vi "Read SubComponent Parameter - Raw.vi"(8 "error in (no error)":errorcluster, 10 "Parameter":string, 11 "1553 SubComponent in":refnum<class "1553 SubComponent.lvclass">) -> (0 "error out":errorcluster, 2 "Raw Data":u64 format="%016x")   [LabVIEW 2020, in "BCI-1553 API.lvlib" / "1553 SubComponent.lvclass"]
doc: "Reads a raw U64 value for a single parameter, as opposed to all the parameters at once."
uses:
  1553 SubComponent.lvclass
  Frames & Messages/TypeDefs/Parameter Table Data.ctl
  Frames & Messages/TypeDefs/Scaling Information.ctl
  1553 SubComponent.lvclass/1553 SubComponent.ctl
  Dependencies/Registry/Registry.lvclass/Registry.ctl
  Dependencies/Registry/Registry.lvclass
  BCI-1553 API.lvlib
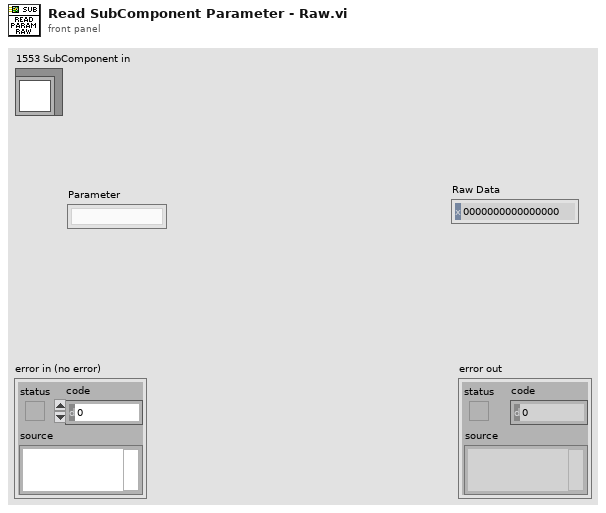
[diagram p1: front panel]
types:
  T1 = typedef "BCI-1553 API.lvlib/Parameter Table Data.ctl" = cluster{"Parameter Name":string, "Base Word":u16, "Address":u16, "Value":u64, "Mask":u16[], "Scaling Info":T2}
  T2 = typedef "BCI-1553 API.lvlib/Scaling Information.ctl" = cluster{"Bit Offset":i32, "Bit Count":i32, "LSB Resolution":dbl, "2's Complement":bool, "Big Endian":bool, "Sign Bit":bool}
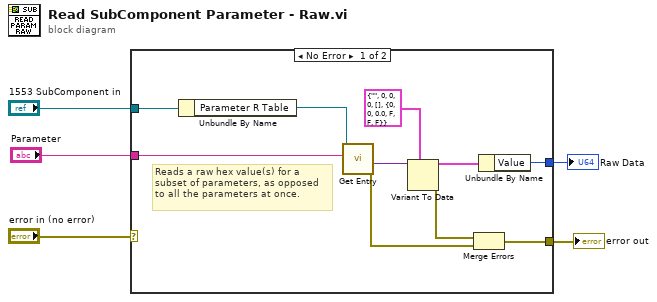
[diagram p0: block diagram]
diagram:
  n1 = case shown="No Error" "error in (no error)" {
    selector: "error in (no error)" -> [_ w16]
    tunnel: [w6 w16] -> w4
    tunnel: "1553 SubComponent in" -> [w15 _]
    tunnel: "Parameter" -> [w13 _]
    tunnel: [w9 _] -> w1
    frame No Error {
      # "Reads a raw hex value(s) for a\nsubset of parameters, as opposed\nto all the parameters at once."
      n2 = Unbundle By Name(w15) -> ("Parameter R Table"=w14:refnum<class "Registry.lvclass">)
      n3 = call "Get Entry.vi"("Key"=w13, "Registry in"=w14) -> ("error out"=w7:errorcluster, "Value"=w11:variant)  [unwired: 6 in, 2 out]
      n4 = Variant To Data(type=T1 {"Parameter Name"="", "Base Word"=0, "Address"=0, "Value"=0, "Mask"=[], "Scaling Info"={"Bit Offset"=0, "Bit Count"=0, "LSB Resolution"=0.0, "2's Complement"=FALSE, "Big Endian"=FALSE, "Sign Bit"=FALSE}} ("Parameter Table Data"), Variant=w11) -> (data=w12:T1, error out=w8:errorcluster)  [unwired: 1 in]
      n5 = Merge Errors(w8, w7) -> (w6:errorcluster)
      n6 = Unbundle By Name(w12) -> ("Value"=w9:u64)
    }
    frame Error {
    }
  }
  "error out" <- w4
  "Raw Data" <- w1
